vi "__2400_set_c_curr.vi"(4 "curr_set(mA)":dbl=0.0004, 7 "GPIB":string="24") -> (0 "error out":errorcluster caption="エラー出力")   [LabVIEW 2017]
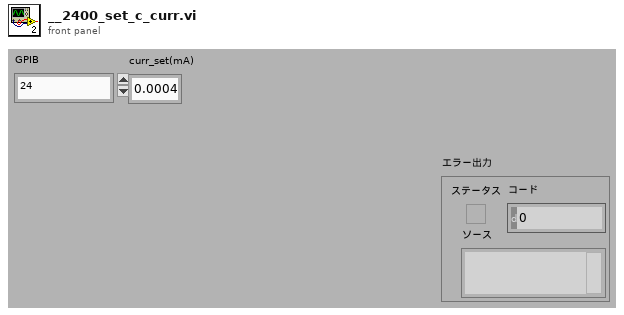
[diagram p1: front panel]
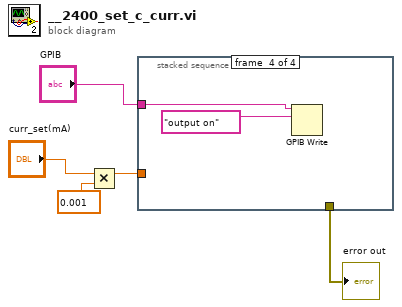
[diagram p0: block diagram]
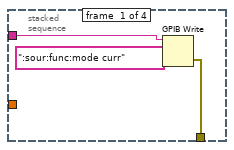
[diagram p2: hidden frame]
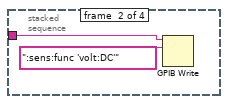
[diagram p3: hidden frame]
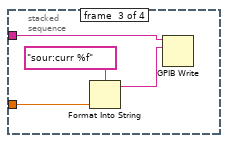
[diagram p4: hidden frame]
diagram:
  n1 = Multiply(x="curr_set(mA)", y=0.001) -> (x*y=w3:dbl)
  n2 = stacked-sequence {
    tunnel: "GPIB" -> [w8 w10 w14 w16]
    tunnel: w3 -> [_ _ w12 _]
    tunnel: [w6 _ _ _] -> w1
    frame #0 {
      n3 = GPIB Write(0:w8, 1:":sour:func:mode curr") -> (6:w6:errorcluster)  [unwired: 3 in, 1 out]
    }
    frame #1 {
      n4 = GPIB Write(0:w10, 1:":sens:func 'volt:DC'") -> ()  [unwired: 3 in, 2 out]
    }
    frame #2 {
      n5 = Format Into String(format string="sour:curr %f", w12) -> (resulting string=w11:string)  [unwired: 2 in, 1 out]
      n6 = GPIB Write(0:w14, 1:w11) -> ()  [unwired: 3 in, 2 out]
    }
    frame #3 {
      n7 = GPIB Write(0:w16, 1:"output on") -> ()  [unwired: 3 in, 2 out]
    }
  }
  "error out" <- w1
